vi "Compile Digital Pattern Gen 1.0 Data.vi"(8 "error in (no error)":errorcluster, 11 "Device Item Ref in":T3 format="%.0x") -> (0 "error out":errorcluster, 1 "bitfile names":string[](array[string]), 2 "Digital Pattern Gens":T1[](array[typedef]), 3 "Device Item Ref out":T3 format="%.0x")   [LabVIEW 2020, in "Engine Simulation Toolkit System Explorer.lvlib"]
uses:
  Engine Simulation Toolkit System Explorer.lvlib
  <vilib>/NI VeriStand/Custom Device API/Custom Device Item Ref.ctl
  Shared/1.0 Digital Pattern Gen Engine Data.ctl
  Shared/1.0 Digital Pattern Gen FIFO Idxs.ctl
  Digital Pattern Find Events Enum.ctl
  Shared/Constants and GUIDs.vi
  <vilib>/NI VeriStand/Custom Device Tools/Custom Device Utility Library/NI VeriStand - Search for Item by GUID.vi
  <vilib>/NI VeriStand/Custom Device Tools/Custom Device Utility Library/Custom Device Utility Library.lvlib
  Shared/Engine Simulation Toolkit Shared.lvlib
  <vilib>/NI VeriStand/Custom Device API/Custom Device API.lvlib
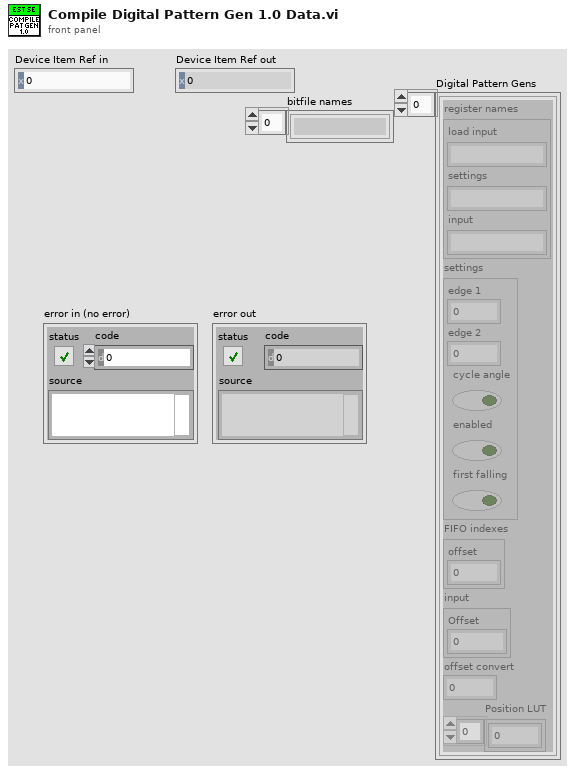
[diagram p1: front panel]
types:
  T1 = typedef "Engine Simulation Toolkit Shared.lvlib/1.0 Digital Pattern Gen Engine Data.ctl" = cluster{"register names":cluster{"load input":string, "settings":string, "input":string}, "settings":cluster{"edge 1":u16, "edge 2":u16, "cycle angle":bool, "enabled":bool, "first falling":bool}, "FIFO indexes":T2, "input":cluster{"Offset":i16}, "offset convert":dbl, "Position LUT":u16[]}
  T2 = typedef "Engine Simulation Toolkit Shared.lvlib/1.0 Digital Pattern Gen FIFO Idxs.ctl" = cluster{"offset":i32}
  T3 = typedef "Custom Device API.lvlib/Custom Device Item Ref.ctl" = u64
  T4 = typedef "Engine Simulation Toolkit Shared.lvlib/Channel.ctl" = cluster{"Name":string, "Units":string, "Default":dbl, "Description":string, "Scalable":bool}
  T5 = typedef "Engine Simulation Toolkit System Explorer.lvlib/Digital Pattern.ctl" = cluster{"Name":string, "Base":T6, "Remove":T7[], "Add":T8[], "FPGA Resource":string}
  T6 = typedef "Engine Simulation Toolkit System Explorer.lvlib/Digital Pattern Base.ctl" = cluster{"Length":dbl, "Teeth":u16, "Width":dbl, "Offset":dbl}
  T7 = typedef "Engine Simulation Toolkit System Explorer.lvlib/Digital Pattern Remove Edge.ctl" = cluster{"Tooth":u16, "Edge":bool}
  T8 = typedef "Engine Simulation Toolkit System Explorer.lvlib/Digital Pattern Add Pulse.ctl" = cluster{"Tooth":u16, "Offset":dbl, "Width":dbl}
  T9 = typedef "Engine Simulation Toolkit System Explorer.lvlib/Digital Pattern Find Events Enum.ctl" = enum16{"Rising Edge", "Falling Edge", "Any Edge", "Center Tooth", "Center Gap"}
  T10 = typedef "Engine Simulation Toolkit System Explorer.lvlib/Digital Pattern Expanded.ctl" = cluster{"X":dbl[], "Y":dbl[]}
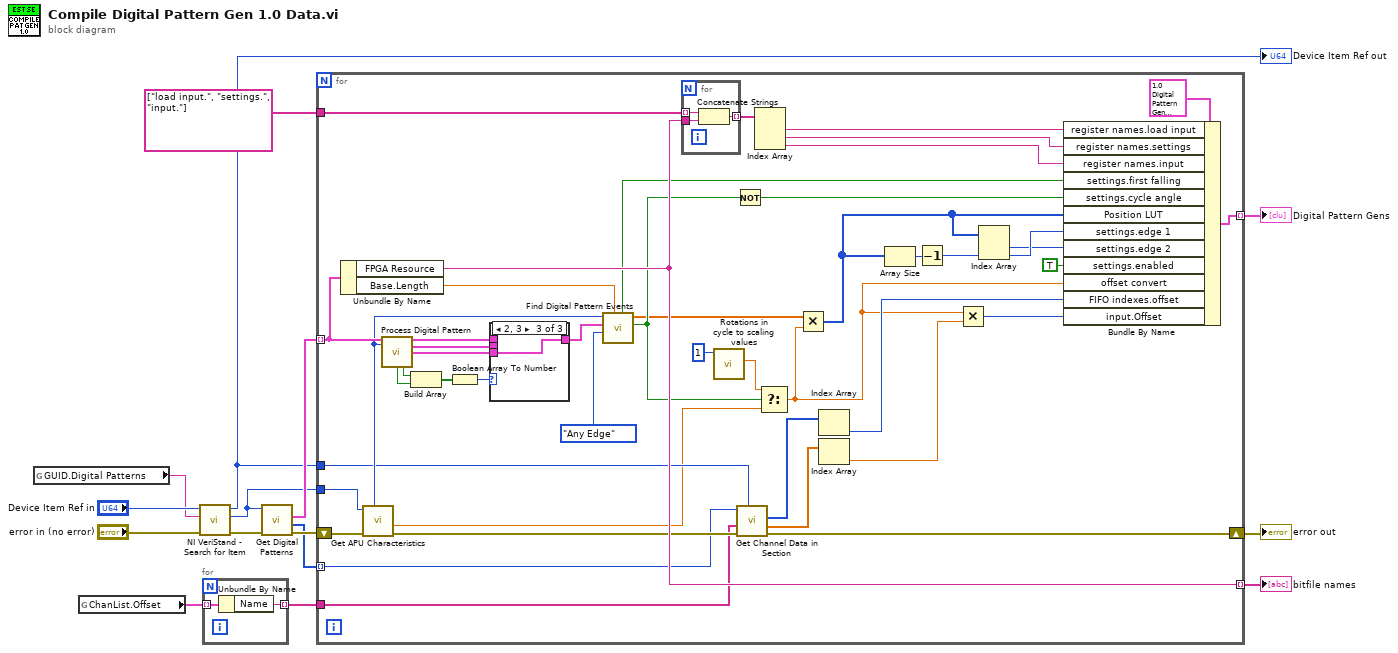
[diagram p0: block diagram]
diagram:
  n1 = global read "Constants and GUIDs.vi" "GUID.Digital Patterns"() -> (w13:string)
  n2 = global read "Constants and GUIDs.vi" "ChanList.Offset"() -> (w2:T4[])
  n3 = call-poly <vilib>:"NI VeriStand - Search for Item.vi"("error in"="error in (no error)", "Item GUID"=w13, "Section Ref in"="Device Item Ref in") -> ("error out"=w12:errorcluster, "Item Ref"=w4:T3, "Section Ref out"=w5:T3)  [unwired: 5 in, 1 out]
  "Device Item Ref out" <- w5
  n4 = for {
    tunnel: [w17] -> w1 mode=indexing
    tunnel: w2 -> [w16] mode=indexing
    n5 = Unbundle By Name(w16) -> ("Name"=w17:string)
  }
  n6 = call "Get Digital Patterns.vi"("error in (no error)"=w12, "Item Ref in"=w4) -> ("error out"=w7:errorcluster, "references"=w3:T3[], "Patterns"=w6:T5[])  [unwired: 7 in]
  n7 = for {
    shift-right: [w39] -> w10
    shift-left: w7 -> [w54]
    tunnel: w6 -> [w52] mode=indexing
    tunnel: string[] ["load input.", "settings.", "input."] -> [w63]
    tunnel: [w58] -> w9 mode=indexing
    tunnel: [w56] -> w8 mode=indexing
    tunnel: w5 -> [w37]
    tunnel: w4 -> [w53]
    tunnel: w3 -> [w38] mode=indexing
    tunnel: w1 -> [w36]
    n8 = Unbundle By Name(w52) -> ("FPGA Resource"=w56:string, "Base.Length"=w50:dbl)
    n9 = call "Get APU Characteristics.vi"("error in (no error)"=w54, "Item Ref in"=w53) -> ("error out"=w47:errorcluster, "angle to u16 scale factor"=w20:dbl, "rotations"=w51:u16)  [unwired: 3 in, 4 out]
    n10 = call "Process Digital Pattern.vi"("EPT Pattern"=w52, "Rotations"=w51) -> ("Base"=w24:T10, 6:"Reduced"=w23:T10, 8:"Final"=w22:T10, 13:"Final"=w27:bool, 14:"Reduced"=w28:bool)  [unwired: 7 in, 2 out]
    n11 = Build Array(w28, w27) -> (w26:bool[])
    n12 = Boolean Array To Number(Boolean array=w26) -> (number=w25:u32)
    n13 = case shown="2, 3" w25 {
      tunnel: w24 -> [w64 _ _]
      tunnel: w23 -> [_ w65 _]
      tunnel: w22 -> [_ _ w66]
      tunnel: [w64 w65 w66] -> w21
      frame 0, Default {
      }
      frame 1 {
      }
      frame 2, 3 {
      }
    }
    n14 = call "Find Digital Pattern Events.vi"("Base.length"=w50, "Event"=Digital_Pattern_Find_Events_Enum."Any Edge", "Pattern"=w21, "Rotations"=w51) -> ("crank angle"=w48:bool, "Locations"=w46:dbl[], "first falling"=w18:bool)  [unwired: 5 in]
    n15 = for {
      tunnel: w56 -> [w69]
      tunnel: w63 -> [w68] mode=indexing
      tunnel: [w67] -> w61 mode=indexing
      n16 = Concatenate Strings(w68, w69) -> (w67:string)
    }
    n17 = call "Rotations in cycle to scaling values.vi"("rotations in a cycle"=u16 1) -> ("angle to u16 scale factor"=w19:dbl)  [unwired: 8 in, 2 out]
    n18 = Not(x=w48) -> (.not. x?=w29:bool)
    n19 = call "Get Channel Data in Section.vi"("Custom device ref"=w37, "error in (no error)"=w47, "Channels"=w36, "Item Ref in"=w38) -> ("error out"=w39:errorcluster, "default values"=w33:dbl[], "FIFO indexes"=w35:i32[])  [unwired: 3 in, 2 out]
    n20 = Index Array(array=w61) -> (element #1=w60:string, element #2=w59:string, element #3=w57:string)  [unwired: 3 in]
    n21 = Select(t=w19, s=w48, f=w20) -> (s? t:f=w31:dbl)
    n22 = Multiply(x=w46, y=w31) -> (x*y=w40:u16[])
    n23 = Index Array(array=w35) -> (element=w34:i32)  [unwired: 1 in]
    n24 = Index Array(array=w33) -> (element=w32:dbl)  [unwired: 1 in]
    n25 = Array Size(array=w40) -> (size(s)=w44:i32)
    n26 = Decrement(x=w44) -> (x-1=w43:i32)
    n27 = Multiply(x=w31, y=w32) -> (x*y=w30:i16)
    n28 = Index Array(array=w40, index #2=w43) -> (element #1=w41:u16, element #2=w42:u16)  [unwired: 1 in]
    n29 = Bundle By Name(cluster=T1 {"register names"={"load input"="", "settings"="", "input"=""}, "settings"={"edge 1"=0, "edge 2"=0, "cycle angle"=FALSE, "enabled"=FALSE, "first falling"=FALSE}, "FIFO indexes"={"offset"=0}, "input"={"Offset"=0}, "offset convert"=0.0, "Position LUT"=[]} ("1.0.0 Digital Pattern Gen"), "register names.load input"=w60, "register names.settings"=w59, "register names.input"=w57, "settings.first falling"=w18, "settings.cycle angle"=w29, "Position LUT"=w40, "settings.edge 1"=w42, "settings.edge 2"=w41, "settings.enabled"=TRUE, "offset convert"=w31, "FIFO indexes.offset"=w34, "input.Offset"=w30) -> (w58:T1)
  }
  "error out" <- w10
  "Digital Pattern Gens" <- w9
  "bitfile names" <- w8
